vi "Gui Interlock Tester-UTF-Test-VI.vi"() -> (3 "Unit Test Framework Results":T1)   [LabVIEW 2018]
doc: "Use this template to create a user-defined test VI. Define your test requirements and wire the results to the <b>Result (Test)</b> control. Do not modify the <b>Unit Test Framework Results</b> indicator."
uses:
  <vilib>/utf/common/utf_test_result_troll.ctl
  <vilib>/utf/common/utf_test_result.ctl
  <vilib>/utf/common/utf_test_result_failure.ctl
  <vilib>/utf/common/utf_test_comparison_operators.ctl
  <vilib>/utf/common/utf_vi_tag.ctl
  <vilib>/utf/NI_UnitTestFramework.lvlib
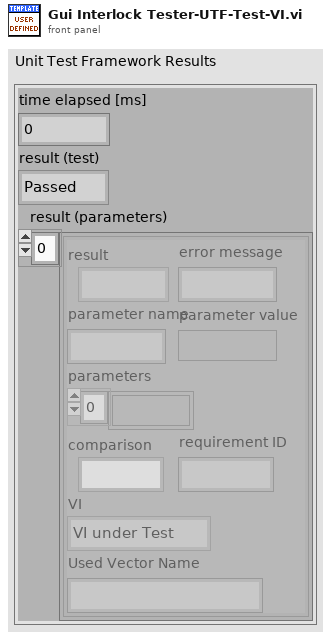
[diagram p1: front panel]
types:
  T1 = typedef "NI_UnitTestFramework.lvlib/utf_test_result_troll.ctl" = cluster{"time elapsed [ms]":u32, "result (test)":T2, "result (parameters)":T3[]}
  T2 = typedef "NI_UnitTestFramework.lvlib/utf_test_result.ctl" = enum16{"Passed", "Failed", "Error", "Skipped", "Not Processed"}
  T3 = typedef "NI_UnitTestFramework.lvlib/utf_test_result_failure.ctl" = cluster{"result":T2, "error message":string, "parameter name":string, "parameter value":variant, "parameters":variant[], "comparison":T4, "requirement ID":string, "VI":T5, "Used Vector Name":string}
  T4 = typedef "NI_UnitTestFramework.lvlib/utf_test_comparison_operators.ctl" = enum16{"=", "!=", ">", ">=", "<", "<=", "range", "symmetric tolerance", "asymmetric tolerance", "string contains", "string not contain", "array size", "string length", "array range", "by element", "array range (limit array)", "user-defined", "array contains", "array not contain", "vector length", "= (elm)", "!= (elm)", "= (case insensitive)", "!= (case insensitive)"}
  T5 = typedef "NI_UnitTestFramework.lvlib/utf_vi_tag.ctl" = enum16{"Setup VI", "VI under Test", "Teardown VI"}
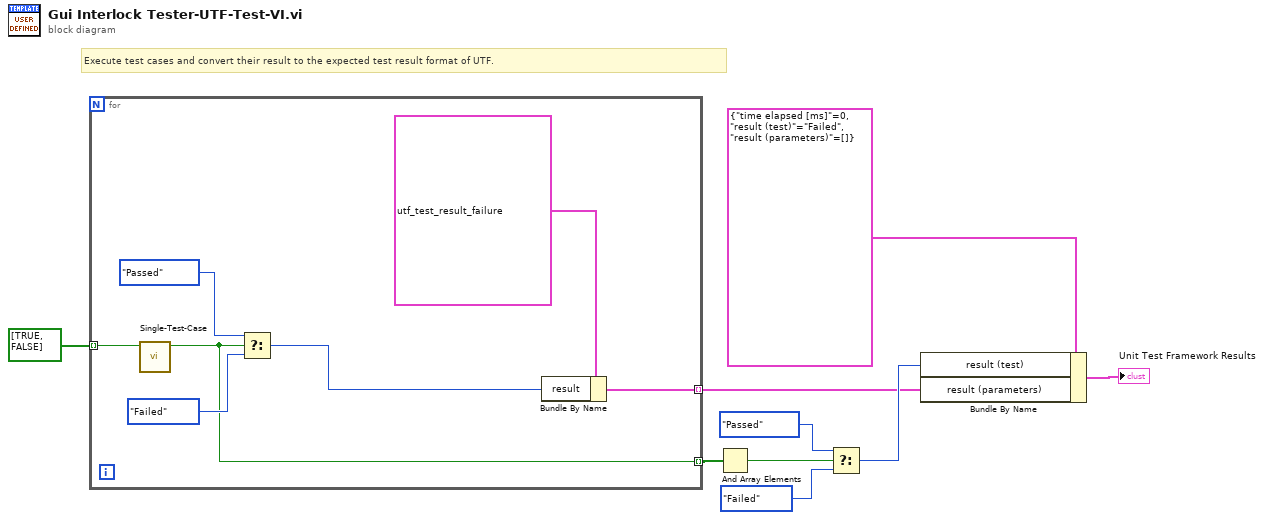
[diagram p0: block diagram]
diagram:
  # "Execute test cases and convert their result to the expected test result format of UTF."
  n1 = for {
    tunnel: bool[] [TRUE, FALSE] -> [w15] mode=indexing
    tunnel: [w11] -> w2 mode=indexing
    tunnel: [w10] -> w7 mode=indexing
    n2 = call "Single-Test-Case.vi"("Power On?"=w15) -> ("Test Case Passed"=w10:bool)  [unwired: 10 in]
    n3 = Select(t=utf_test_result."Passed" ("result"), s=w10, f=utf_test_result."Failed" ("result")) -> (s? t:f=w14:T2)
    n4 = Bundle By Name(cluster=T3 {"result"=enum."Not Processed", "error message"="", "parameter name"="", "parameter value"=variant, "parameters"=[], "comparison"=enum."=", "requirement ID"="", "VI"=enum."VI under Test", "Used Vector Name"=""} ("Unit Test Framework - result (parameters)"), "result"=w14) -> (w11:T3)
  }
  n5 = And Array Elements(Boolean array=w7) -> (logical AND=w4:bool)
  n6 = Select(t=utf_test_result."Passed" ("result"), s=w4, f=utf_test_result."Failed" ("result")) -> (s? t:f=w3:T2)
  n7 = Bundle By Name(cluster=T1 {"time elapsed [ms]"=0, "result (test)"=enum."Failed", "result (parameters)"=[]} ("Unit Test Framework - Result"), "result (test)"=w3, "result (parameters)"=w2) -> (→"Unit Test Framework Results":T1)
